vi "Check Status.vi"(8 "error in (no error)":errorcluster, 11 "Spectrometer iHR320 in":refnum<class "Spectrometer iHR320.lvclass">) -> (0 "error out":errorcluster, 1 "Status":string, 2 "Ready?":bool, 3 "Spectrometer iHR320 out":refnum<class "Spectrometer iHR320.lvclass">)   [LabVIEW 2009, in "Spectrometer iHR320.lvclass"]
doc: "(Dynamic) Check if the instrument is powered on and update its member fields with the instrument's current status. Optionally return a text status message."
uses:
  Spectrometer iHR320.lvclass
  Utility Classes/Scannable/Scannable.lvclass
  Spectrometer iHR320.lvclass/Spectrometer iHR320.ctl
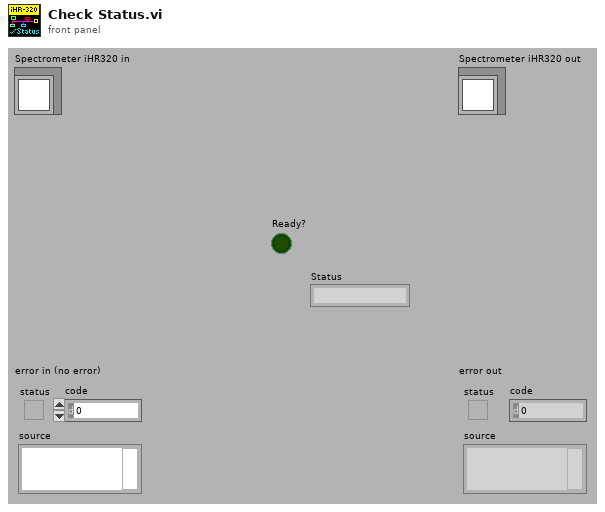
[diagram p1: front panel]
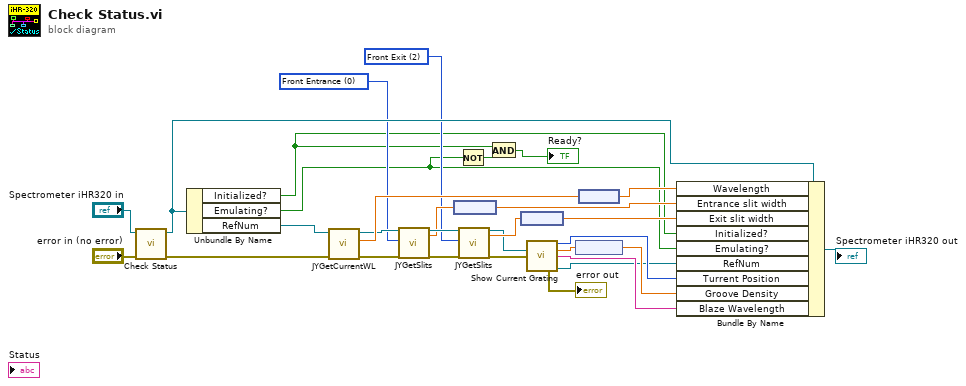
[diagram p0: block diagram]
diagram:
  w5 = u16 2 items=["Front Entrance", "Side Entrance", "Front Exit", "Side Exit", "First Intermediate", "Second Intermediate"] ("Slit")
  w22 = u16 0 items=["Front Entrance", "Side Entrance", "Front Exit", "Side Exit", "First Intermediate", "Second Intermediate"] ("Slit")
  n1 = call-parent "Check Status.vi"("error in (no error)"="error in (no error)", "Instrument in"="Spectrometer iHR320 in") -> ("error out"=w27:errorcluster, "Instrument out"=w26:refnum<class "Spectrometer iHR320.lvclass">)  [unwired: 6 in, 2 out]
  n2 = Unbundle By Name(w26) -> ("Initialized?"=w1:bool, "Emulating?"=w2:bool, "RefNum"=w28:refnum<k7>)
  n3 = call "JYGetCurrentWL.vi"("error in (no error)"=w27, "JYMONOLib.IJYMonoReqd In"=w28) -> ("error out"=w21:errorcluster, "Current WL"=w25:dbl, "JYMONOLib.IJYMonoReqd Out"=w23:refnum<k7>)  [unwired: 6 in, 1 out]
  n4 = call "JYGetSlits.vi"("MonoRefNum IN"=w23, "Slit"=w22, "error in (no error)"=w21) -> ("MonoRefNum Out"=w19:refnum<k7>, "Slit Width"=w18:dbl, "error out"=w20:errorcluster)  [unwired: 13 in, 1 out]
  n5 = node(w18) -> (w17:dbl[unit])
  n6 = Not(x=w2) -> (.not. x?=w3:bool)
  n7 = call "JYGetSlits.vi"("MonoRefNum IN"=w19, "Slit"=w5, "error in (no error)"=w20) -> ("MonoRefNum Out"=w14:refnum<k7>, "Slit Width"=w16:dbl, "error out"=w13:errorcluster)  [unwired: 13 in, 1 out]
  n8 = And(x=w1, y=w3) -> (x .and. y?=→"Ready?":bool)
  n9 = node(w16) -> (w15:dbl[unit])
  n10 = call "Show Current Grating.vi"("JYMONOLib.IJYMonoReqd  in"=w14, "error in (no error)"=w13) -> ("Grating Index"=w12:i32, "Current Grating"=w11:dbl, "Current Blaze"=w9:string, "error out"=→"error out":errorcluster, "JYMONOLib.IJYMonoReqd Out"=w7:refnum<k7>)  [unwired: 5 in, 4 out]
  n11 = node(w11) -> (w10:dbl[unit])
  n12 = node(w25) -> (w24:dbl[unit])
  n13 = Bundle By Name(cluster=w26, "Wavelength"=w24, "Entrance slit width"=w17, "Exit slit width"=w15, "Initialized?"=w1, "Emulating?"=w2, "RefNum"=w7, "Turrent Position"=w12, "Groove Density"=w10, "Blaze Wavelength"=w9) -> (→"Spectrometer iHR320 out":refnum<class "Spectrometer iHR320.lvclass">)
